vi "Settings Dialog.vi"(8 "error in (no error)":errorcluster, 11 "Settings in":T1={"Hardware Configuration"={"DAQmx Channel"="", "Max Input"=10.0, "Min Input"=-10.0, "Sample Rate"=1000.0, "DAQmx Task"=""}, "Logging Configuration"={"Log File Base Path"=path "", "TDMS File Reference"=refnum, "Samples to Save"=0, "InterRecording Delay"=0.0}}) -> (0 "error out":errorcluster, 1 "Cancelled?":bool=TRUE, 2 "UI Refresh Needed?":bool, 3 "Settings out":T1={"Hardware Configuration"={"DAQmx Channel"="", "Max Input"=10.0, "Min Input"=-10.0, "Sample Rate"=1000.0, "DAQmx Task"=""}, "Logging Configuration"={"Log File Base Path"=path "C:/Users/jpassiak/Documents/LabVIEW Data/Logged Data.tdms", "TDMS File Reference"=refnum, "Samples to Save"=0, "InterRecording Delay"=0.0}})   [LabVIEW 2014, in "Settings.lvlib"]
doc: "Dialog for selecting user specified settings."
uses:
  Settings.lvlib
  Settings.ctl
  Acquisition/Hardware Configuration.ctl
  Logging/Logging Configuration.ctl
  <vilib>/Utility/xml.llb/Write to XML File(string).vi
  Acquisition/Acquisition.lvlib
  Logging/Logging.lvlib
panel:
  in  "Interval Between Recordings (sec)":dbl format="%#_13g"
  in  "Length of Recordings (sec)":dbl=500.0 min=1.0
  in  "Sample Rate":dbl=1000.0
  in  "Minimum Input":dbl=-10.0
  in  "Maximum Input":dbl=10.0
  in  "DAQmx Channel":tag="Dev1/ai0"
  in  "Log File Path":path
  in  "Cancel Button":bool
  in  "OK Button":bool
  # "Acquisition"
  # "Non visible portion of dialog (needed for connector pane)."
  # "Timer Function"
  # "Logging"
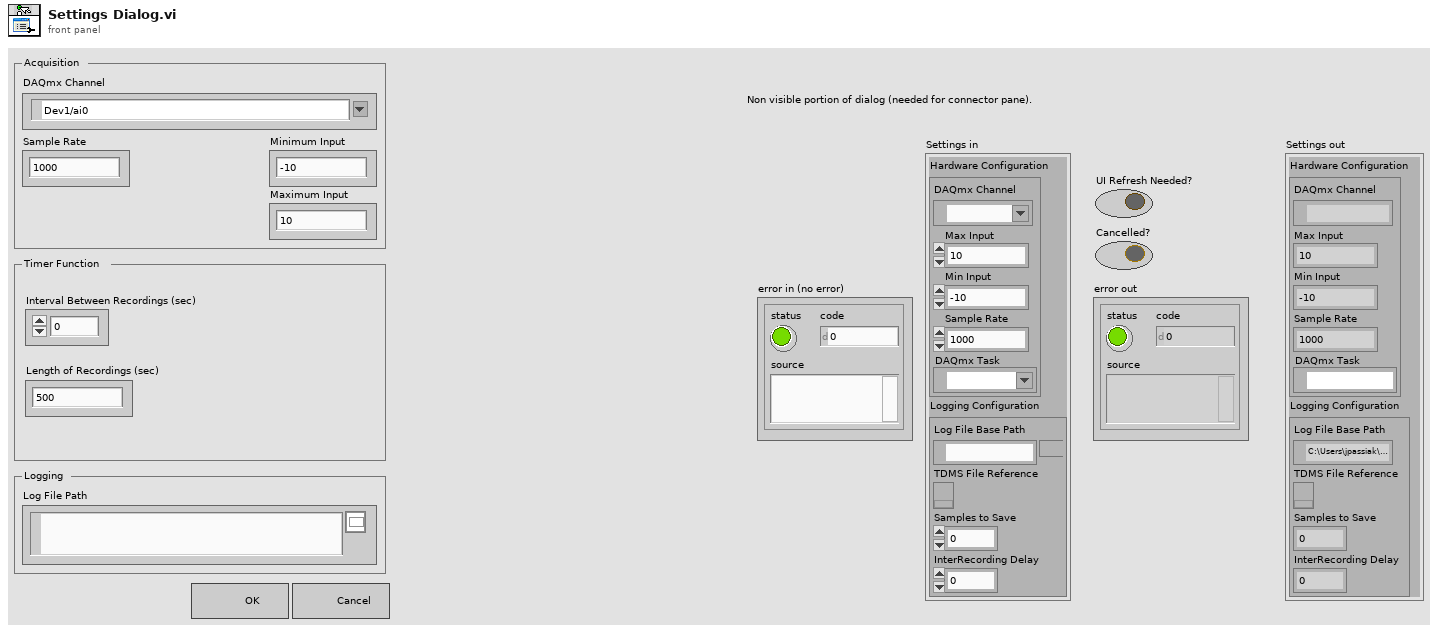
[diagram p1: front panel]
types:
  T1 = typedef "Settings.lvlib/Settings.ctl" = cluster{"Hardware Configuration":T2, "Logging Configuration":T3}
  T2 = typedef "Acquisition.lvlib/Hardware Configuration.ctl" = cluster{"DAQmx Channel":tag, "Max Input":dbl, "Min Input":dbl, "Sample Rate":dbl, "DAQmx Task":refnum<k21>}
  T3 = typedef "Logging.lvlib/Logging Configuration.ctl" = cluster{"Log File Base Path":path, "TDMS File Reference":refnum<k34>, "Samples to Save":u32, "InterRecording Delay":dbl}
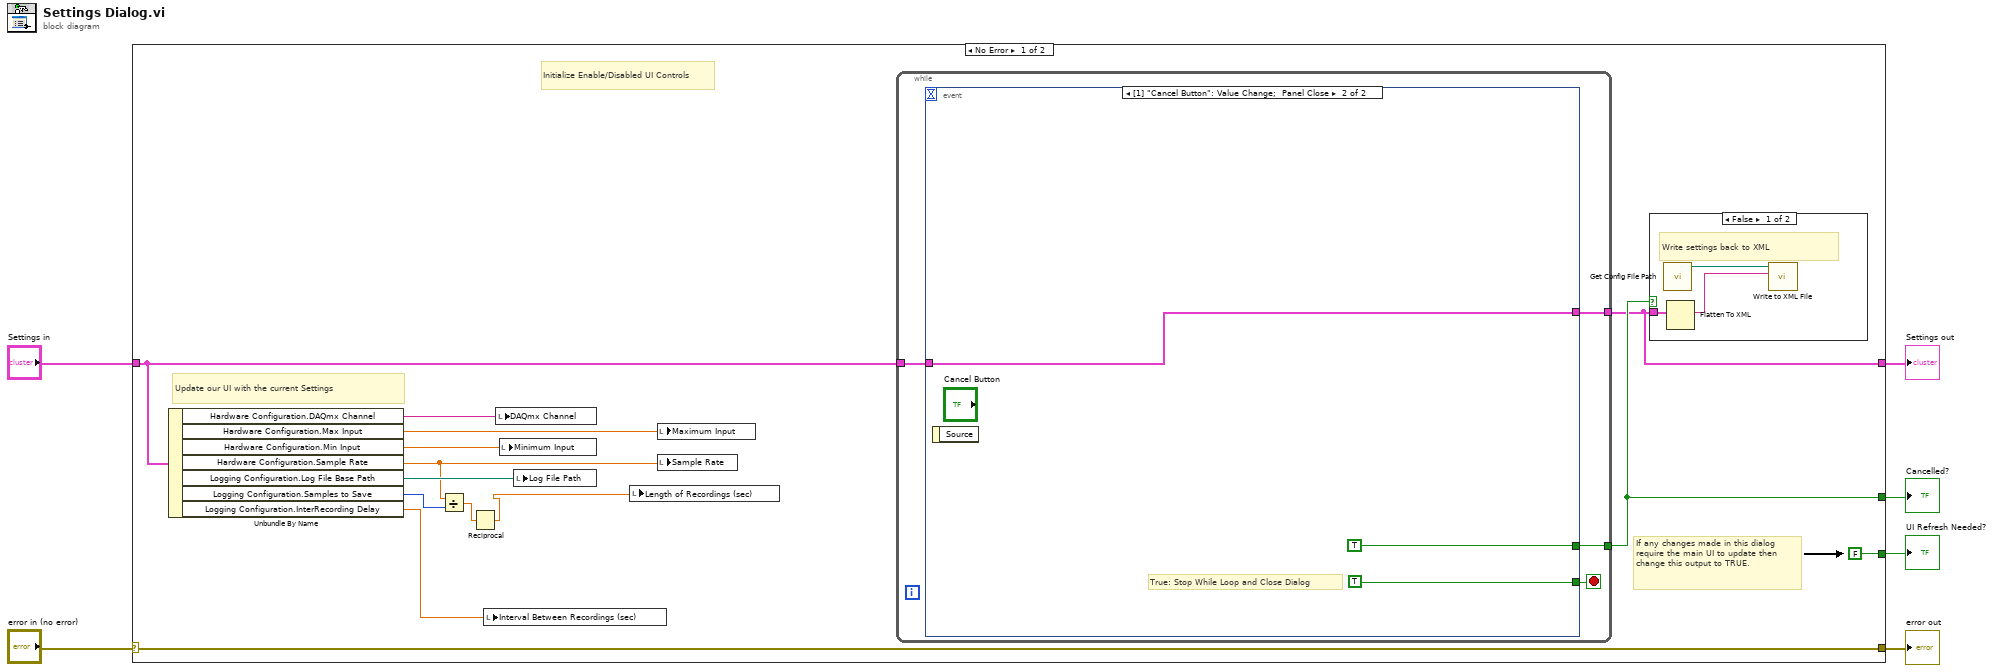
[diagram p0: block diagram]
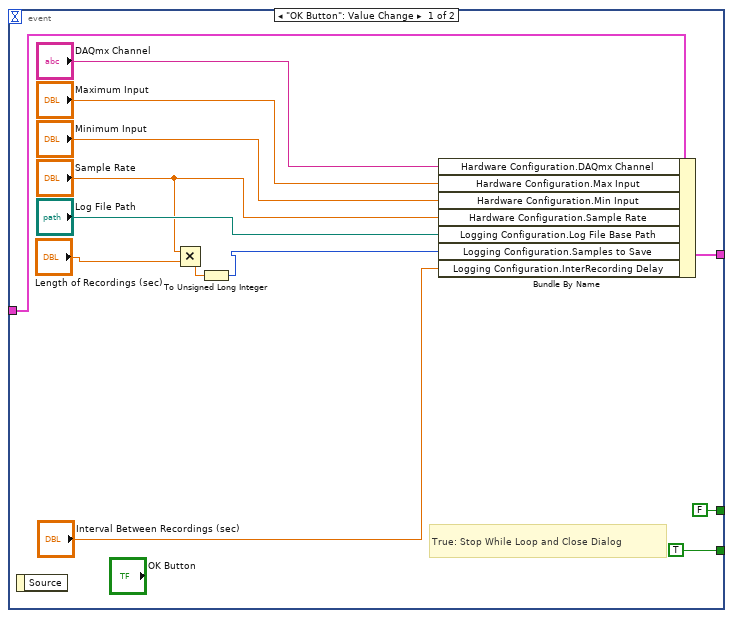
[diagram p2: hidden frame]
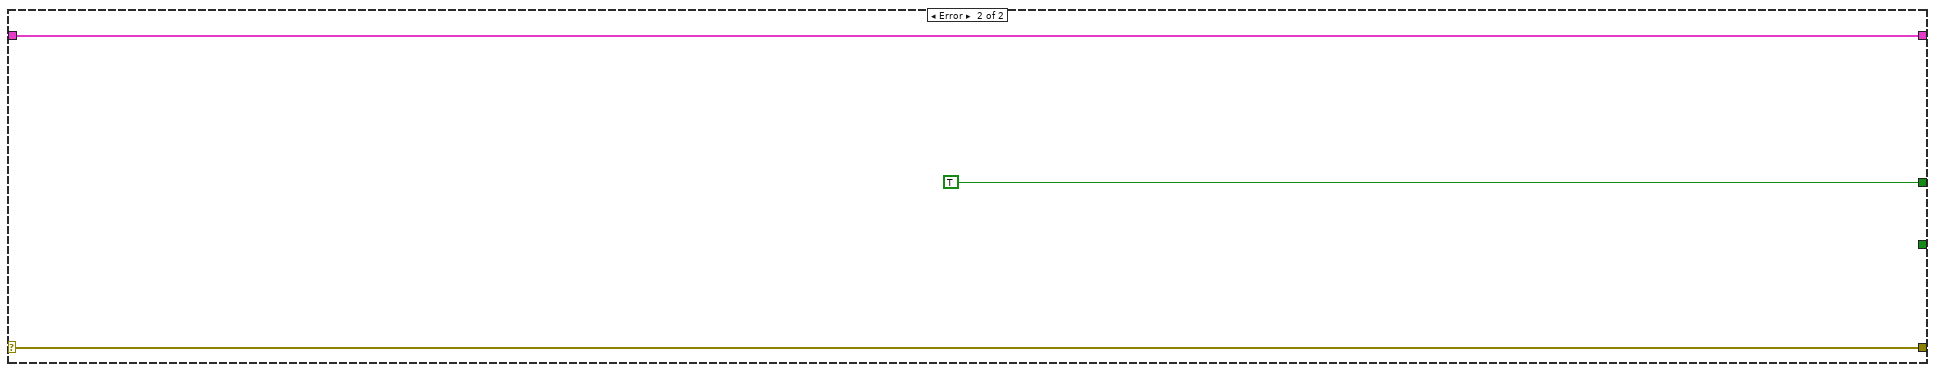
[diagram p4: hidden frame]
diagram:
  n1 = case shown="No Error" "error in (no error)" {
    selector: "error in (no error)" -> [w20 w46]
    tunnel: [w20 w46] -> w6
    tunnel: "Settings in" -> [w12 w45]
    tunnel: [w17 w45] -> w1
    tunnel: [FALSE ("UI Refresh Needed?") _] -> w4
    tunnel: [w18 TRUE ("UI Refresh Needed?")] -> w3
    frame No Error {
      # "Update our UI with the current Settings"
      # "Initialize Enable/Disabled UI Controls"
      # "If any changes made in this dialog require the main UI to update then change this output to TRUE."
      n2 = Unbundle By Name(w12) -> ("Hardware Configuration.DAQmx Channel"=w14:tag, "Hardware Configuration.Max Input"=w15:dbl, "Hardware Configuration.Min Input"=w16:dbl, "Hardware Configuration.Sample Rate"=w9:dbl, "Logging Configuration.Log File Base Path"=w13:path, "Logging Configuration.Samples to Save"=w10:u32, "Logging Configuration.InterRecording Delay"=w11:dbl)
      n3 = Divide(x=w9, y=w10) -> (x/y=w7:dbl)
      n4 = Reciprocal(x=w7) -> (1/x=w8:dbl)
      n5 = local write "Interval Between Recordings (sec)"(w11) -> ()
      n6 = local write "DAQmx Channel"(w14) -> ()
      n7 = local write "Minimum Input"(w16) -> ()
      n8 = local write "Log File Path"(w13) -> ()
      n9 = local write "Length of Recordings (sec)"(w8) -> ()
      n10 = local write "Maximum Input"(w15) -> ()
      n11 = local write "Sample Rate"(w9) -> ()
      n12 = while {
        tunnel: [w24] -> w18
        tunnel: [w23] -> w17
        tunnel: w12 -> [w22]
        stop <- w21 stop-if-true
        n13 = event shown="[1] \"Cancel Button\": Value Change;  Panel Close" {
          selector: _ -> [_ _]
          dyn-events: _ -> [_ _]
          timeout: _ -> [_ _]
          tunnel: [w35 w40] -> w23
          tunnel: w22 -> [w34 w40]
          tunnel: [FALSE ("UI Refresh Needed?") TRUE ("UI Refresh Needed?")] -> w24
          tunnel: [TRUE TRUE] -> w21
          event "OK Button": Value Change {
            # "True: Stop While Loop and Close Dialog"
            n14 = event-data() -> ()  [unwired: 1 in, 1 out]
            n15 = Multiply(x="Sample Rate", y="Length of Recordings (sec)") -> (x*y=w27:dbl)
            n16 = To Unsigned Long Integer(number=w27) -> (unsigned 32bit integer=w28:u32)
            n17 = Bundle By Name(cluster=w34, "Hardware Configuration.DAQmx Channel"="DAQmx Channel", "Hardware Configuration.Max Input"="Maximum Input", "Hardware Configuration.Min Input"="Minimum Input", "Hardware Configuration.Sample Rate"="Sample Rate", "Logging Configuration.Log File Base Path"="Log File Path", "Logging Configuration.Samples to Save"=w28, "Logging Configuration.InterRecording Delay"="Interval Between Recordings (sec)") -> (w35:T1)
          }
          event "Cancel Button": Value Change; Panel Close {
            # "True: Stop While Loop and Close Dialog"
            n18 = event-data() -> ()  [unwired: 1 in, 1 out]
          }
        }
      }
      n19 = case shown="False" w18 {
        tunnel: w17 -> [w42 _]
        frame False {
          # "Write settings back to XML"
          n20 = call "Get Config File Path.vi"() -> ("XML File Path"=w43:path)  [unwired: 10 in, 1 out]
          n21 = Flatten To XML(anything=w42) -> (xml string=w41:string)
          n22 = call-poly <vilib>:"Write to XML File.vi"("XML Input"=w41, "XML File Path"=w43) -> ()  [unwired: 7 in, 3 out]
        }
        frame True {
        }
      }
    }
    frame Error {
    }
  }
  "UI Refresh Needed?" <- w4
  "error out" <- w6
  "Settings out" <- w1
  "Cancelled?" <- w3
